vi "Write Z_Source.vi"(8 "error in (no error)":errorcluster, 10 "Z_Source":T1, 11 "Z_HSw in":refnum<class "Z_OnSw.lvclass">) -> (0 "error out":errorcluster, 3 "Z_HSw out":refnum<class "Z_OnSw.lvclass">)   [LabVIEW 2019, in "Z_OnSw.lvclass"]
uses:
  Z_OnSw.lvclass
  Z_source.ctl
  Z_OnSw.lvclass/Z_OnSw.ctl
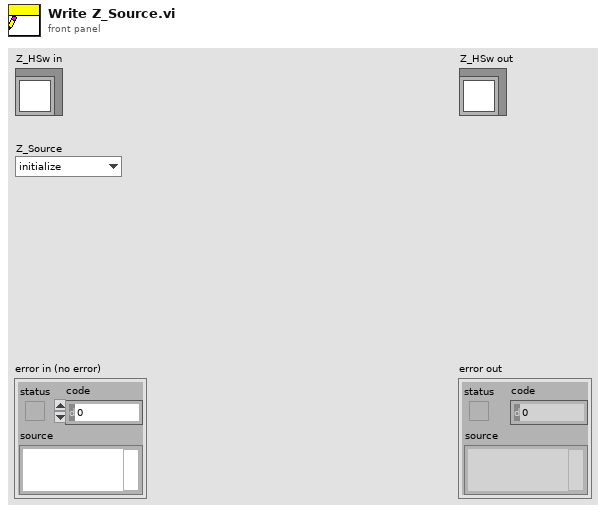
[diagram p1: front panel]
types:
  T1 = typedef "Z_source.ctl" = enum8{"initialize", "local disabled", "local hand", "hand", "auto", "dist"}
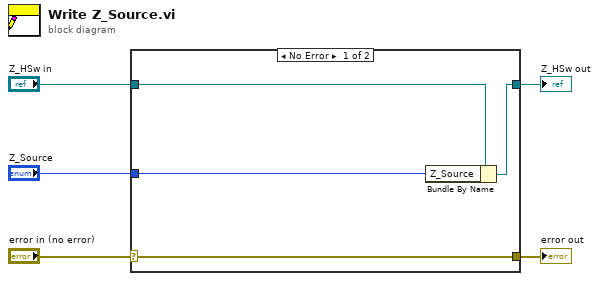
[diagram p0: block diagram]
diagram:
  n1 = case shown="No Error" "error in (no error)" {
    selector: "error in (no error)" -> [w9 w10]
    tunnel: [w9 w10] -> w4
    tunnel: [w7 w11] -> w2
    tunnel: "Z_HSw in" -> [w8 w11]
    tunnel: "Z_Source" -> [w6 _]
    frame No Error {
      n2 = Bundle By Name(cluster=w8, "Z_Source"=w6) -> (w7:refnum<class "Z_OnSw.lvclass">)
    }
    frame Error {
    }
  }
  "error out" <- w4
  "Z_HSw out" <- w2
